vi "Configure List Parameters.vi"(0 "VISA resource name":refnum<visa-resource-name>, 1 "Step Number (1)":i32=1 min=1 max=150 step=1 format="%#.0p", 5 "Step Voltage (1.000)":dbl=1.0 min=0.0 max=150.0 step=1.0 format="%.3f", 7 "Step Current (1.0000)":dbl=1.0 min=0.0 max=25.0 step=1.0 format="%.4f", 9 "Step Time (1)":dbl=1.0 min=0.1 max=9999.9 step=0.1 format="%.1f", 11 "error in (no error)":errorcluster) -> (4 "VISA resource name out":refnum<visa-resource-name>, 15 "error out":errorcluster)   [LabVIEW 2021, in "BK Precision 9200 Series.lvlib"]
doc: "Configures the step voltage, current, and time of a list step.\n\nNote: Changes will not be saved until <b>Save Recall List Program.vi</b> is ran.\nThe steps must be configured sequentially. If a step is skipped with programmed parameters, the list program will stop running when it reaches that step."
uses:
  <instrlib>/BK Precision 9200 Series/BK Precision 9200 Series.lvlib
panel:
  # "s"
  # "A"
  # "V"
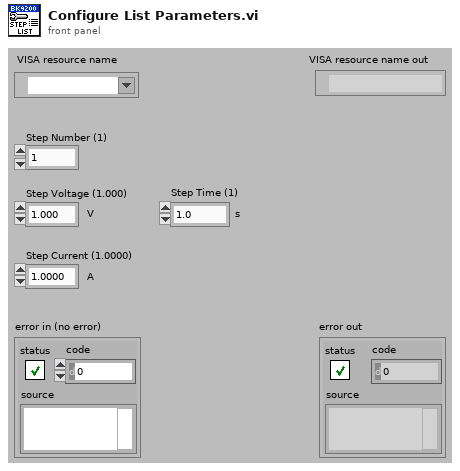
[diagram p1: front panel]
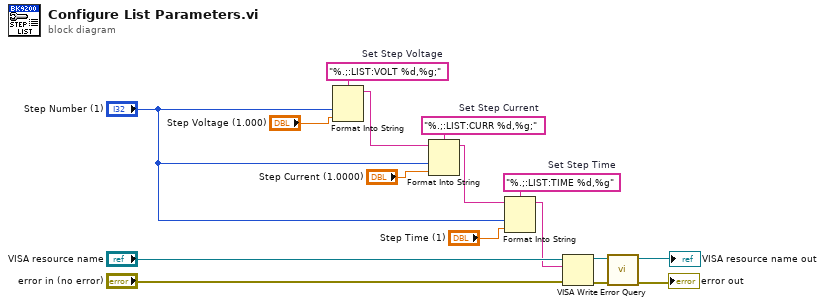
[diagram p0: block diagram]
diagram:
  w10 = "%.;:LIST:VOLT %d,%g;"  # Set Step Voltage
  w11 = "%.;:LIST:CURR %d,%g;"  # Set Step Current
  w16 = "%.;:LIST:TIME %d,%g"  # Set Step Time
  n1 = Format Into String(format string=w10, "Step Number (1)", "Step Voltage (1.000)") -> (resulting string=w9:string)  [unwired: 2 in, 1 out]
  n2 = Format Into String(format string=w11, initial string=w9, "Step Number (1)", "Step Current (1.0000)") -> (resulting string=w8:string)  [unwired: 1 in, 1 out]
  n3 = Format Into String(format string=w16, initial string=w8, "Step Number (1)", "Step Time (1)") -> (resulting string=w1:string)  [unwired: 1 in, 1 out]
  n4 = VISA Write(VISA resource name="VISA resource name", write buffer=w1, error in (no error)="error in (no error)") -> (VISA resource name out=w15:refnum<visa-resource-name>, error out=w14:errorcluster)  [unwired: 1 out]
  n5 = call <instrlib>:"Error Query.vi"("error in (no error)"=w14, "VISA resource name"=w15) -> ("error out"=→"error out":errorcluster, "VISA resource name out"=→"VISA resource name out":refnum<visa-resource-name>)  [unwired: 6 in, 2 out]
